vi "Ver 1.3.vi"() -> ()   [LabVIEW 2015]
uses:
  <instrlib>/Keithley 622x LV 2009/Configure/Source/Typedefs/KE622x -- Current Range.ctl
  <instrlib>/Keithley 622x LV 2009/Configure/Source/Typedefs/KE622x -- Current Ranges.ctl
  <instrlib>/Keithley 622x LV 2009/Typedefs/KE622x -- On Off Control.ctl
  <instrlib>/Keithley 622x LV 2009/Utility/Typedefs/KE622x -- Instrument Type.ctl
  <instrlib>/Keithley 622x LV 2009/Configure/Source/Typedefs/KE622x -- Voltage Limit.ctl
  <instrlib>/Keithley 2000/Public/Configure/Configure DC Volts.vi
  <instrlib>/Keithley 2000/Keithley 2000.lvlib
  <instrlib>/Keithley 622x LV 2009/Keithley 622x.lvlib
panel:
  out "XY Graph":cluster{u32[], dbl[]}(graph)
  out "Measurement":dbl
  out "T0":u32
  out "LIMIT":bool
  out "LIMIT":bool
  out "Error Code":string
  in  "Comments":string
  out "file":refnum<file>
  out "2000":refnum<visa-resource-name>
  out "6221":refnum<visa-resource-name>
  in  "Step  (A)":dbl=5e-05 format="%#_3p"
  in  "Stop\ncurrent (A)":dbl=0.002 format="%#_6p"
  in  "Start \ncurrent (A)":dbl=0.001 format="%#_6p"
  in  "Check For SCPI Errors? (T)":bool=TRUE
  out "Interlock Tripped?":bool
  out "Compliance?":bool
  in  "Turn Off Output \nIf Compliance?":bool=TRUE
  in  "Turning ON/OFF\ncurrent output":T1=enum."On"
  in  "Range Selection":T2={"Auto Range?"=TRUE, "Man / Selected\nRange"=enum."2nA"}
  # "FILE CONFIGURATION"
  # "ADMIN PANEL"
  # "KEITHLEY 6221 CONFIGURATION (ADMIN ONLY)"
  # "I don't know what the hell it is,\njust don't touch it"
  # "START, STOP, STEP, CONFIGURATION"
  # "IF ON"
  # "Compliance = Limiting output voltage\nThis switch determines if we want to switch \noff the current output if wee exceed compliance"
  # "There is a safe switch at \nthe back of the instrument \nThis indicator shows if it is on"
  # "You have hit a damn jackpot \nby exceeding the limited voltage\nCongrats"
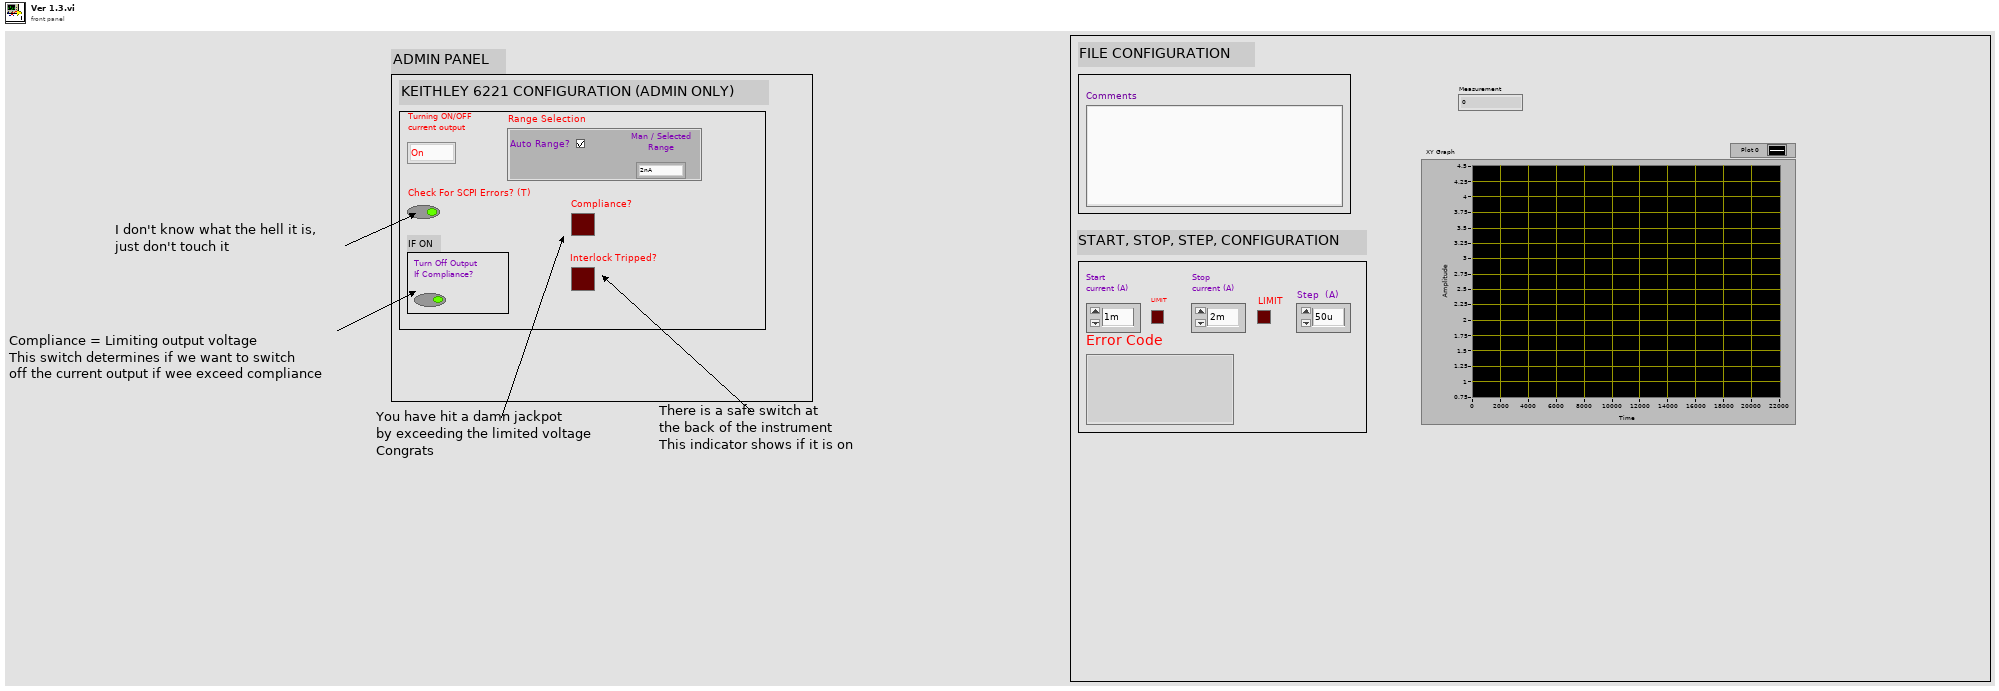
[diagram p1: front panel]
types:
  T1 = typedef "Keithley 622x.lvlib/KE622x -- On Off Control.ctl" = enum16{"Off", "On"}
  T2 = typedef "Keithley 622x.lvlib/KE622x -- Current Range.ctl" = cluster{"Auto Range?":bool, "Man / Selected\nRange":T3}
  T3 = typedef "Keithley 622x.lvlib/KE622x -- Current Ranges.ctl" = enum16{"2nA", "20nA", "200nA", "2uA", "20uA", "200uA", "2mA", "20mA", "100mA"}
  T4 = typedef "Keithley 622x.lvlib/KE622x -- Voltage Limit.ctl" = dbl
  T5 = typedef "Keithley 622x.lvlib/KE622x -- Instrument Type.ctl" = enum16{"KE6220", "KE6221"}
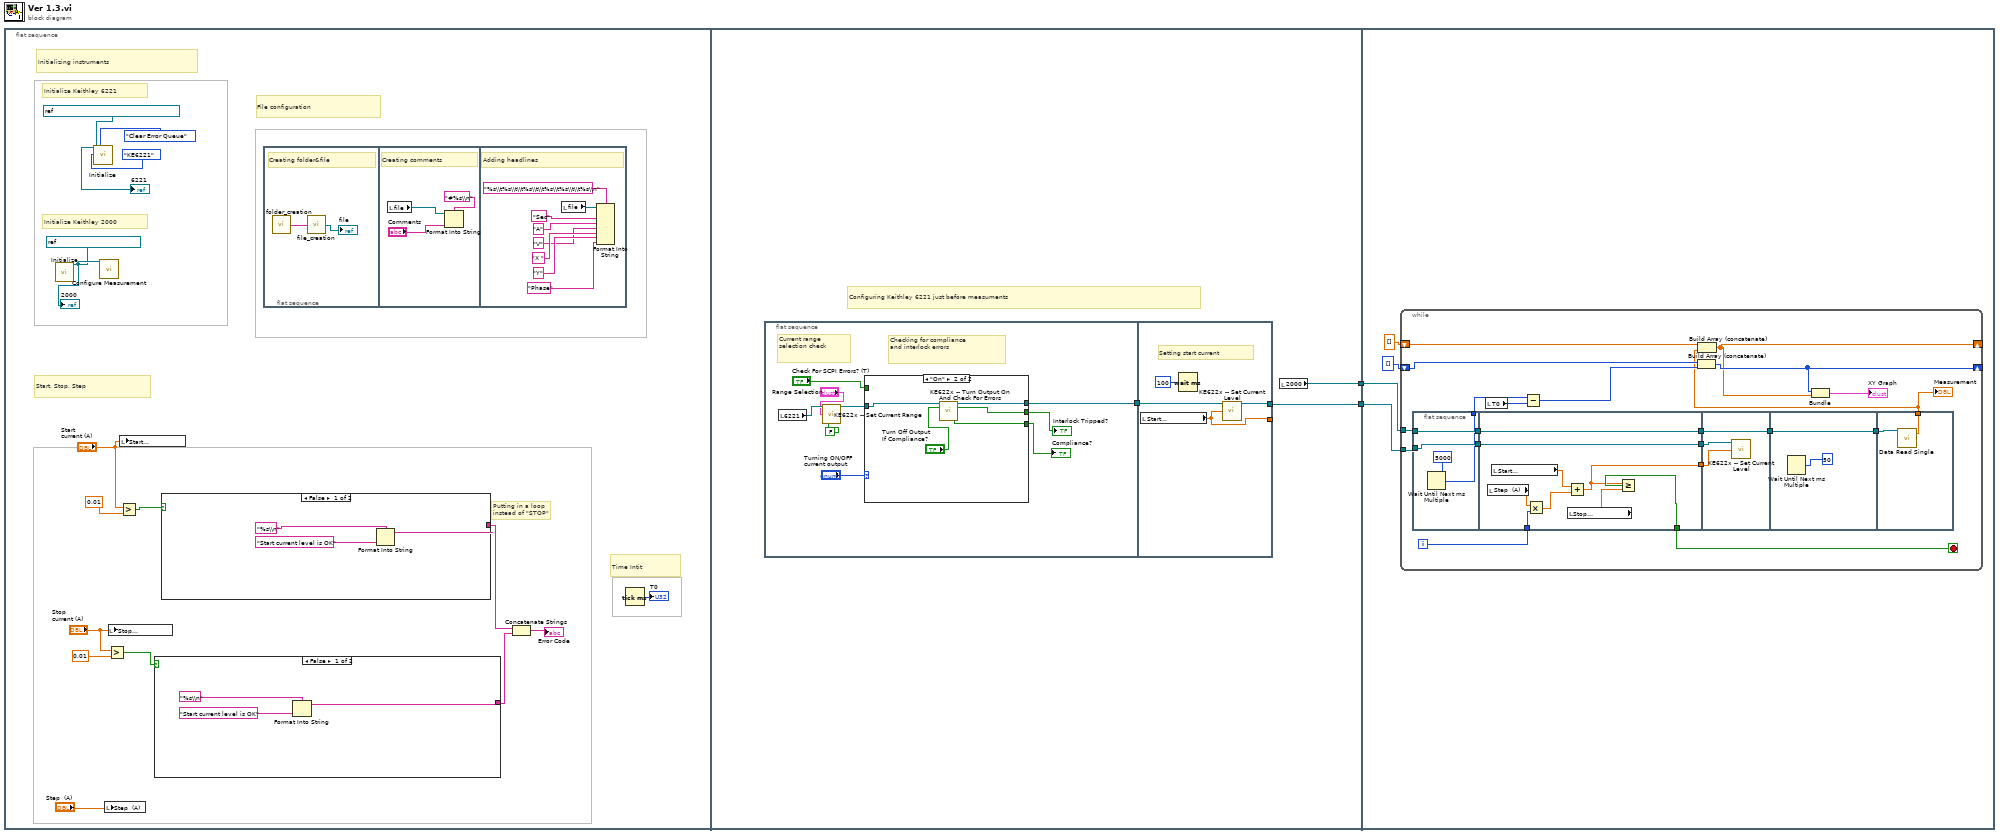
[diagram p0: block diagram]
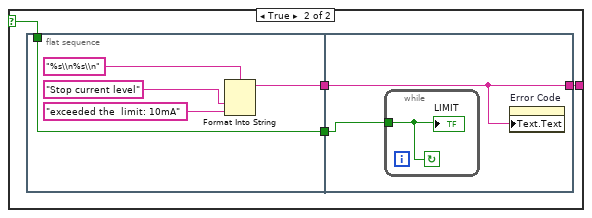
[diagram p2: hidden frame]
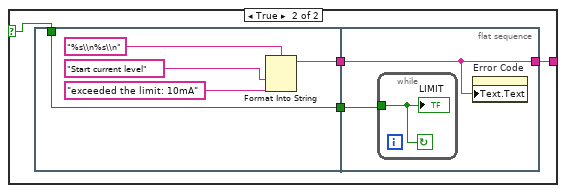
[diagram p3: hidden frame]
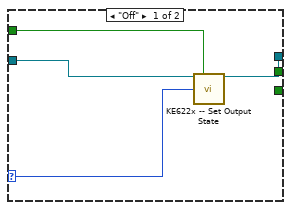
[diagram p4: hidden frame]
diagram:
  n1 = flat-sequence {
    tunnel: [w64] -> w2
    tunnel: [w63] -> w1
    tunnel: w2 -> [w89]
    tunnel: w1 -> [w88]
    frame #0 {
      # "Time Intit"
      # "Putting in a loop \ninstead of \"STOP\""
      # "Start, Stop, Step"
      # "Initializing instruments"
      # "File configuration"
      # "Initialize Keithley 2000"
      # "Initialize Keithley 6221"
      n2 = call <instrlib>:"Initialize.vi"("VISA resource name"=refnum<visa-resource-name> "KEITHLEY_MULTIMETER") -> ("VISA resource name out"=w15:refnum<visa-resource-name>)  [unwired: 17 in, 1 out]
      "2000" <- w15
      n3 = call <instrlib>:"Initialize.vi"("VISA resource name"=refnum<visa-resource-name> "KEITHLEY_DC_AC_CURRENT_SOURCE", "Error Queue Option"=enum16{"Clear Error Queue", "Error Query"}."Clear Error Queue", "Instrument Type"=KE622x_--_Instrument_Type."KE6221") -> ("VISA resource name out"=→"6221":refnum<visa-resource-name>)  [unwired: 11 in, 1 out]
      n4 = call-poly <instrlib>:"Configure Measurement.vi"("VISA resource name"=w15) -> ()  [unwired: 17 in, 2 out]
      n5 = local write "Step  (A)"("Step  (A)") -> ()
      n6 = Greater?(x="Stop\ncurrent (A)", y=T4 0.01) -> (0:w7:bool)
      n7 = local write "Stop\ncurrent (A)"("Stop\ncurrent (A)") -> ()
      n8 = local write "Start \ncurrent (A)"("Start \ncurrent (A)") -> ()
      n9 = Greater?(x="Start \ncurrent (A)", y=T4 0.01) -> (0:w8:bool)
      n10 = case shown="False" w7 {
        selector: w7 -> [_ w23]
        tunnel: [w20 w26] -> w5
        frame False {
          n11 = Format Into String(format string="%s\\n", "Start current level is OK" ("false string")) -> (resulting string=w20:string)  [unwired: 2 in, 1 out]
        }
        frame True {
          n12 = flat-sequence {
            tunnel: [w28] -> w25
            tunnel: [w27] -> w24
            tunnel: w23 -> [w27]
            tunnel: [w32] -> w26
            tunnel: w25 -> [w32]
            tunnel: w24 -> [w33]
            frame #0 {
              n13 = Format Into String(format string="%s\\n%s\\n", "Stop current level" ("String"), "exceeded the  limit: 10mA" ("input 2")) -> (resulting string=w28:string)  [unwired: 2 in, 1 out]
            }
            frame #1 {
              n14 = while {
                tunnel: w33 -> [w34]
                stop <- w34 continue-if-true
                "LIMIT" <- w34
              }
              n15 = property on="Error Code" class="Str"("Text.Text"=w32) -> ()  [unwired: 2 in, 2 out]
            }
          }
        }
      }
      n16 = case shown="False" w8 {
        selector: w8 -> [_ w39]
        tunnel: [w35 w41] -> w6
        frame False {
          n17 = Format Into String(format string="%s\\n", "Start current level is OK" ("false string")) -> (resulting string=w35:string)  [unwired: 2 in, 1 out]
        }
        frame True {
          n18 = flat-sequence {
            tunnel: [w43] -> w40
            tunnel: w39 -> [w42]
            tunnel: [w42] -> w38
            tunnel: [w47] -> w41
            tunnel: w40 -> [w47]
            tunnel: w38 -> [w48]
            frame #0 {
              n19 = Format Into String(format string="%s\\n%s\\n", "Start current level" ("String"), "exceeded the limit: 10mA" ("input 2")) -> (resulting string=w43:string)  [unwired: 2 in, 1 out]
            }
            frame #1 {
              n20 = while {
                tunnel: w48 -> [w49]
                stop <- w49 continue-if-true
                "LIMIT" <- w49
              }
              n21 = property on="Error Code" class="Str"("Text.Text"=w47) -> ()  [unwired: 2 in, 2 out]
            }
          }
        }
      }
      n22 = flat-sequence {
        frame #0 {
          # "Creating folder&file"
          n23 = call "folder_creation.vi"() -> ("String"=w51:string)
          n24 = call "file_creation.vi"("String"=w51) -> ("refnum out"=→"file":refnum<file>)
        }
        frame #1 {
          # "Creating comments"
          n25 = local read "file"() -> (w52:refnum<file>)
          n26 = Format Into String(format string="#%s\\n", initial string=w52, "Comments") -> ()  [unwired: 1 in, 2 out]
        }
        frame #2 {
          # "Adding headlines"
          n27 = local read "file"() -> (w62:refnum<file>)
          n28 = Format Into String(format string="%s\\t%s\\t\\t%s\\t\\t%s\\t%s\\t\\t%s\\n", initial string=w62, "Sec" ("input 1"), "A" ("input 2"), "V" ("input 3"), "X " ("input 3"), "Y" ("input 3"), "Phase" ("input 3")) -> ()  [unwired: 1 in, 2 out]
        }
      }
      n29 = Concatenate Strings(w6, w5) -> (→"Error Code":string)
      n30 = Tick Count (ms)() -> (millisecond timer value=→"T0":u32)
    }
    frame #1 {
      # "Configuring Keithley 6221 just before measuments"
      n31 = flat-sequence {
        tunnel: [w66] -> w65
        tunnel: [w84] -> _
        tunnel: [w86] -> w63
        tunnel: w65 -> [w85]
        frame #0 {
          # "Current range \nselection check"
          # "Checking for compliance\nand interlock errors"
          n32 = local read "6221"() -> (w69:refnum<visa-resource-name>)
          n33 = call <instrlib>:"KE622x -- Set Current Range.vi"("Resource In"=w69, "Current Range In"="Range Selection", "Read Back Set Values? (T)"=FALSE) -> ("Resource Out (dupl)"=w74:refnum<visa-resource-name>)  [unwired: 10 in, 2 out]
          n34 = case shown="\"On\"" "Turning ON/OFF\ncurrent output" {
            selector: "Turning ON/OFF\ncurrent output" -> [w78 _]
            tunnel: [_ w82] -> w72
            tunnel: [_ w81] -> w73
            tunnel: "Check For SCPI Errors? (T)" -> [w77 _]
            tunnel: w74 -> [w75 w80]
            tunnel: [w76 w79] -> w66
            frame "Off" {
              n35 = call <instrlib>:"KE622x -- Set Output State.vi"("Resource In"=w75, "Check For SCPI Errors? (T)"=w77, "Output State"=w78) -> ("Resource Out (dupl)"=w76:refnum<visa-resource-name>)  [unwired: 11 in, 1 out]
            }
            frame "On" {
              n36 = call <instrlib>:"KE622x -- Turn Output On And Check For Errors.vi"("Resource In"=w80, "Turn Off Output If Compliance?"="Turn Off Output \nIf Compliance?") -> ("Resource Out (dupl)"=w79:refnum<visa-resource-name>, "Interlock Tripped?"=w82:bool, "Compliance?"=w81:bool)  [unwired: 10 in, 1 out]
            }
          }
          "Interlock Tripped?" <- w72
          "Compliance?" <- w73
        }
        frame #1 {
          # "Setting start current"
          n37 = local read "Start \ncurrent (A)"() -> (w84:dbl)
          n38 = Wait (ms)(milliseconds to wait=u32 100) -> ()  [unwired: 1 out]
          n39 = call <instrlib>:"KE622x -- Set Current Level.vi"("Resource In"=w85, "Current Level (A) In"=w84) -> ("Resource Out (dupl)"=w86:refnum<visa-resource-name>)  [unwired: 12 in, 1 out]
        }
      }
      n40 = local read "2000"() -> (w64:refnum<visa-resource-name>)
    }
    frame #2 {
      n41 = while {
        shift-right: [w92] -> _
        shift-left: dbl[] [] -> [w110]
        shift-right: [w93] -> _
        shift-left: i32[] [] -> [w109]
        tunnel: w89 -> [w106]
        tunnel: w88 -> [w104]
        i -> [w100]
        stop <- w99 stop-if-true
        n42 = flat-sequence {
          tunnel: w106 -> [w115]
          tunnel: [w115] -> w105
          tunnel: w104 -> [w114]
          tunnel: [w114] -> w103
          tunnel: [w112] -> w102
          tunnel: [w124] -> w98
          tunnel: w105 -> [w124]
          tunnel: w103 -> [w119]
          tunnel: w100 -> [w121]
          tunnel: [w117] -> w99
          tunnel: [w116] -> w96
          tunnel: [w119] -> w95
          tunnel: w98 -> [w127]
          tunnel: [w127] -> w97
          tunnel: w96 -> [w126]
          tunnel: w95 -> [w125]
          tunnel: w97 -> [w129]
          tunnel: [w129] -> w101
          tunnel: w101 -> [w131]
          tunnel: [w130] -> w94
          frame #0 {
            n43 = Wait Until Next ms Multiple(millisecond multiple=u32 5000) -> (millisecond timer value=w112:u32)
          }
          frame #1 {
            n44 = local read "Step  (A)"() -> (w122:dbl)
            n45 = local read "Start \ncurrent (A)"() -> (w123:dbl)
            n46 = Multiply(x=w122, y=w121) -> (x*y=w120:dbl)
            n47 = local read "Stop\ncurrent (A)"() -> (w118:dbl)
            n48 = Add(x=w123, y=w120) -> (x+y=w116:dbl)
            n49 = Greater Or Equal?(x=w116, y=w118) -> (x >= y?=w117:bool)
          }
          frame #2 {
            n50 = call <instrlib>:"KE622x -- Set Current Level.vi"("Resource In"=w125, "Current Level (A) In"=w126) -> ()  [unwired: 12 in, 2 out]
          }
          frame #3 {
            n51 = Wait Until Next ms Multiple(millisecond multiple=u32 50) -> ()  [unwired: 1 out]
          }
          frame #4 {
            n52 = call <instrlib>:"Data Read Single.vi"("VISA resource name"=w131) -> ("Measurement"=w130:dbl)  [unwired: 14 in, 4 out]
          }
        }
        n53 = local read "T0"() -> (w108:u32)
        n54 = Subtract(x=w102, y=w108) -> (x-y=w107:u32)
        n55 = Build Array (concatenate)(w109, w107) -> (w93:u32[])
        n56 = Build Array (concatenate)(w110, w94) -> (w92:dbl[])
        n57 = Bundle(w93, w92) -> (→"XY Graph":cluster{u32[], dbl[]})  [unwired: 1 in]
        "Measurement" <- w94
      }
    }
  }
